vi "Configure.vi"(8 "error in (no error)":errorcluster, 11 "TomoConversion in":refnum<class "TomoConversion.lvclass">) -> (0 "error out":errorcluster, 2 "cancelled?":bool, 3 "TomoConversion out":refnum<class "TomoConversion.lvclass">)   [LabVIEW 2012, in "TomoConversion.lvclass"]
doc: "The configure method configures the details for the RabbitMQ connection. \n\nIn the derived class, make a call to the parent for setting these parameters."
uses:
  TomoConversion.lvclass
  <vilib>/Utility/miscctls.llb/LVPointTypeDef.ctl
  TomoConversion.lvclass/TomoConversion.ctl
  <vilib>/Distrio/Murmex/Murmex/Murmex.lvclass
panel:
  in  "button::cancel":bool
  in  "button::configuremurmex":bool
  in  "button::ok":bool
  in  "auxiliary director path":path
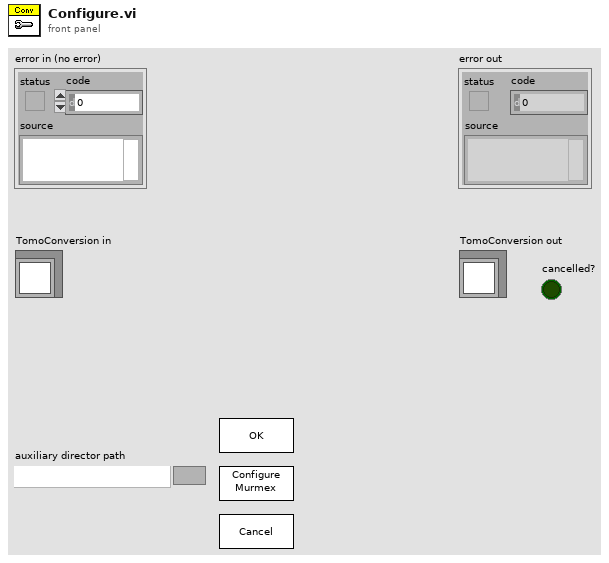
[diagram p1: front panel]
types:
  T1 = typedef "LVPointTypeDef.ctl" = cluster{"Horizontal":i16, "Vertical":i16}
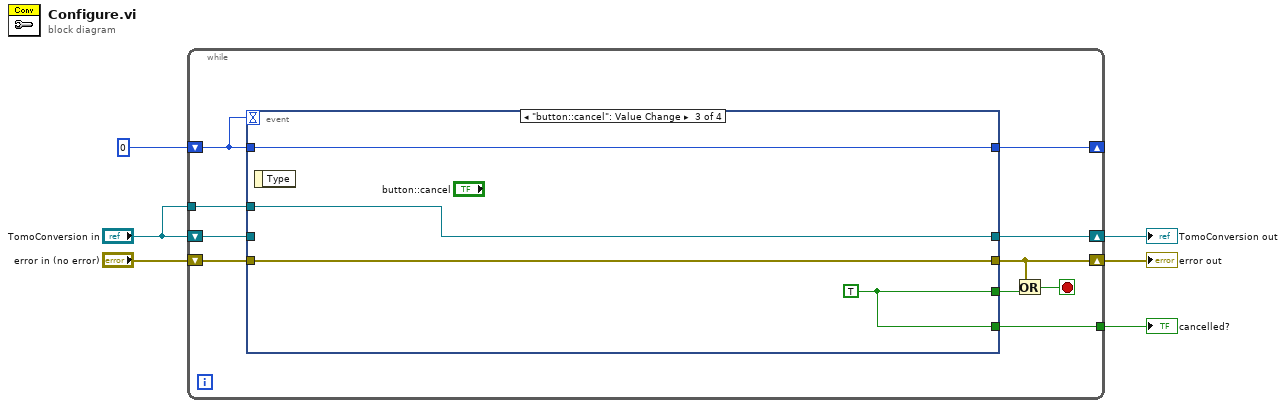
[diagram p0: block diagram]
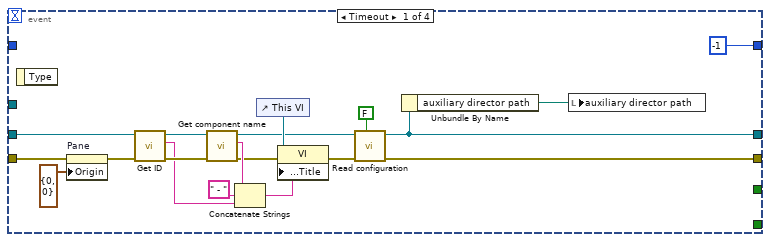
[diagram p2: hidden frame]
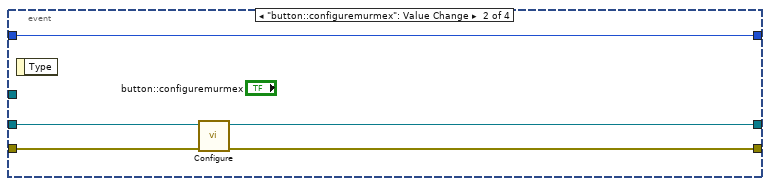
[diagram p3: hidden frame]
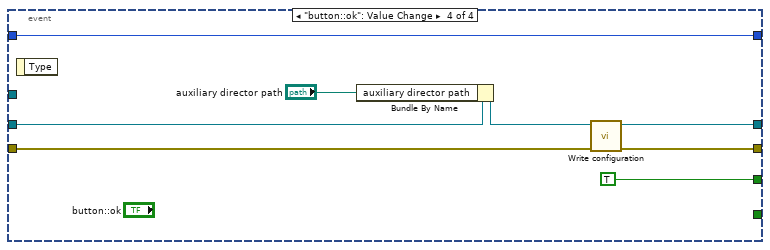
[diagram p4: hidden frame]
diagram:
  n1 = while {
    shift-right: [w11] -> _
    shift-left: 0 -> [w16]
    shift-right: [w12] -> w1
    shift-left: "TomoConversion in" -> [w14]
    shift-right: [w9] -> w2
    shift-left: "error in (no error)" -> [w13]
    tunnel: "TomoConversion in" -> [w15]
    tunnel: [w10] -> w3
    stop <- w7 stop-if-true
    n2 = event shown="[2] \"button::cancel\": Value Change" {
      selector: _ -> [_ _ _ _]
      dyn-events: _ -> [_ _ _ _]
      timeout: w16 -> [_ _ _ _]
      tunnel: w16 -> [_ w36 w41 w45]
      tunnel: w15 -> [_ _ w43 _]
      tunnel: w14 -> [w32 w39 _ w52]
      tunnel: w13 -> [w35 w40 w44 w49]
      tunnel: [w20 w37 w44 w48] -> w9
      tunnel: [w19 w38 w43 w50] -> w12
      tunnel: [-1 w36 w41 w45] -> w11
      tunnel: [_ _ w42 TRUE] -> w8
      tunnel: [_ _ w42 _] -> w10
      event Timeout {
        n3 = event-data() -> ()  [unwired: 1 in, 1 out]
        n4 = property on="Pane" class="Pane"(error in=w35, "Origin"=T1 {"Horizontal"=0, "Vertical"=0}) -> (error out=w33:errorcluster)  [unwired: 1 in, 1 out]
        n5 = call <vilib>:"Get ID.vi"("error in (no error)"=w33, "Murmex in"=w32) -> ("error out"=w30:errorcluster, "component id"=w28:string, "Murmex out"=w31:refnum<class "TomoConversion.lvclass">)  [unwired: 7 in]
        n6 = call <vilib>:"Get component name.vi"("error in (no error)"=w30, "Murmex in"=w31) -> ("error out"=w26:errorcluster, "component name"=w29:string, "Murmex out"=w22:refnum<class "TomoConversion.lvclass">)  [unwired: 7 in]
        n7 = Concatenate Strings(w29, " - " ("string"), w28) -> (w24:string)
        n8 = control-ref of="This VI"() -> (w25:refnum<vi>)
        n9 = property class="VI"(reference=w25, error in=w26, "Front Panel.Title"=w24) -> (error out=w23:errorcluster)  [unwired: 1 out]
        n10 = call-dynamic "Read configuration.vi"("force loading?"=FALSE, "error in (no error)"=w23, "TomoConversion in"=w22) -> ("error out"=w20:errorcluster, "TomoConversion out"=w19:refnum<class "TomoConversion.lvclass">)  [unwired: 7 in]
        n11 = Unbundle By Name(w19) -> ("auxiliary director path"=w18:path)
        n12 = local write "auxiliary director path"(w18) -> ()
      }
      event "button::configuremurmex": Value Change {
        n13 = event-data() -> ()  [unwired: 1 in, 1 out]
        n14 = call-parent "Configure.vi"("error in (no error)"=w40, "Murmex in"=w39) -> ("error out"=w37:errorcluster, "Murmex out"=w38:refnum<class "TomoConversion.lvclass">)  [unwired: 7 in, 1 out]
      }
      event "button::cancel": Value Change {
        w42 = TRUE
        n15 = event-data() -> ()  [unwired: 1 in, 1 out]
      }
      event "button::ok": Value Change {
        n16 = event-data() -> ()  [unwired: 1 in, 1 out]
        n17 = Bundle By Name(cluster=w52, "auxiliary director path"="auxiliary director path") -> (w51:refnum<class "TomoConversion.lvclass">)
        n18 = call-dynamic "Write configuration.vi"("error in (no error)"=w49, "TomoConversion in"=w51) -> ("error out"=w48:errorcluster, "TomoConversion out"=w50:refnum<class "TomoConversion.lvclass">)  [unwired: 8 in]
      }
    }
    n19 = Or(x=w9, y=w8) -> (x .or. y?=w7:bool)
  }
  "error out" <- w2
  "TomoConversion out" <- w1
  "cancelled?" <- w3
